vi "GEOM_ReadDetector.vi"(6 "override format":string, 8 "error in (no error)":errorcluster, 9 "detectors path":path=path "/home/ArcVIEW/Modules/Geometry/database", 10 "Detector Name":string, 11 "database path":path=path "/home/ArcVIEW/Modules/Geometry/database") -> (0 "error out":errorcluster, 2 "Detector":T6 {"ReadModes"."amplifiers"."fliped" items=["none", "horizontal", "vertical"]; "ReadModes"."amplifiers"."type" items=["LL", "LR", "UL", "UR"]}, 3 "file path out":path=path "/home/ArcVIEW/Modules/Geometry/database/TYPES/Hawaii-II_4ch.chp", 5 "ydata":i32, 7 "xdata":i32)   [LabVIEW 2016]
uses:
  GEOM_ReadMode.ctl
  GEOM_Amplifier.ctl
  GEOM_AmpType.ctl
  GEOM_ROI.ctl
  GEOM_Coords.ctl
panel:
  in  "ReadMode":T1 {"amplifiers"."fliped" items=["none", "horizontal", "vertical"]; "amplifiers"."type" items=["LL", "LR", "UL", "UR"]}
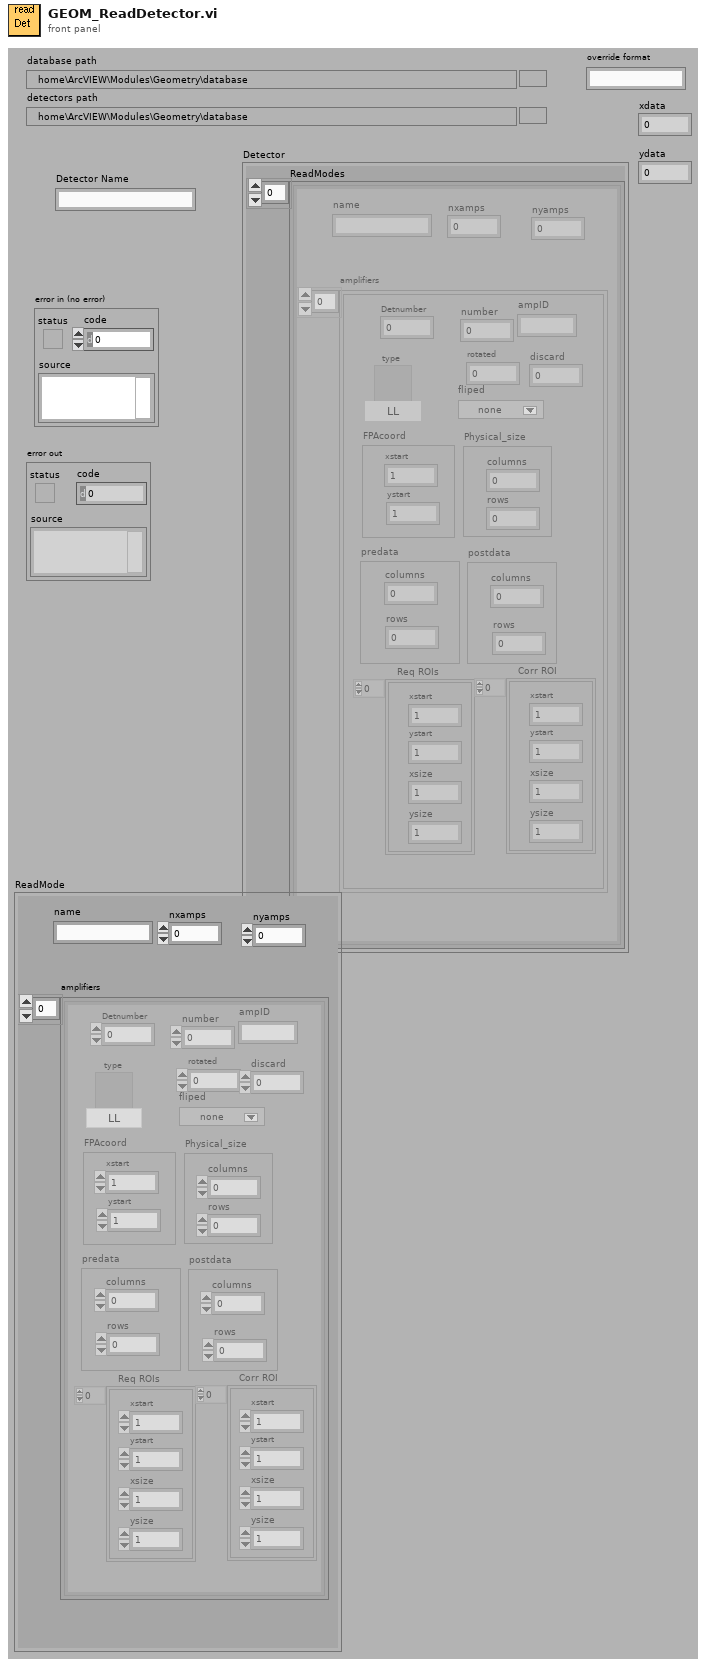
[diagram p1: front panel]
types:
  T1 = typedef "GEOM_ReadMode.ctl" = cluster{"name":string, "amplifiers":T2[], "nxamps":i32, "nyamps":i32}
  T2 = typedef "GEOM_Amplifier.ctl" = cluster{"number":i32, "type":T3, "rotated":i16, "fliped":u16, "FPAcoord":cluster{"xstart":i32, "ystart":i32}, "Physical_size":cluster{"columns":i32, "rows":i32}, "predata":cluster{"columns":i32, "rows":i32}, "postdata":cluster{"columns":i32, "rows":i32}, "Req ROIs":T4, "Corr ROI":T4, "Detnumber":i32, "ampID":string, "discard":i32}
  T3 = typedef "GEOM_AmpType.ctl" = u16
  T4 = typedef "GEOM_ROI.ctl" = T5[]
  T5 = typedef "GEOM_Coords.ctl" = cluster{"xstart":u32, "ystart":u32, "xsize":u32, "ysize":u32}
  T6 = cluster{"name":string, "Info":string[][], "ReadModes":T1[]}
  T7 = cluster{"Detector Name":string, "Info":string[][], "ReadModes":T1[]}
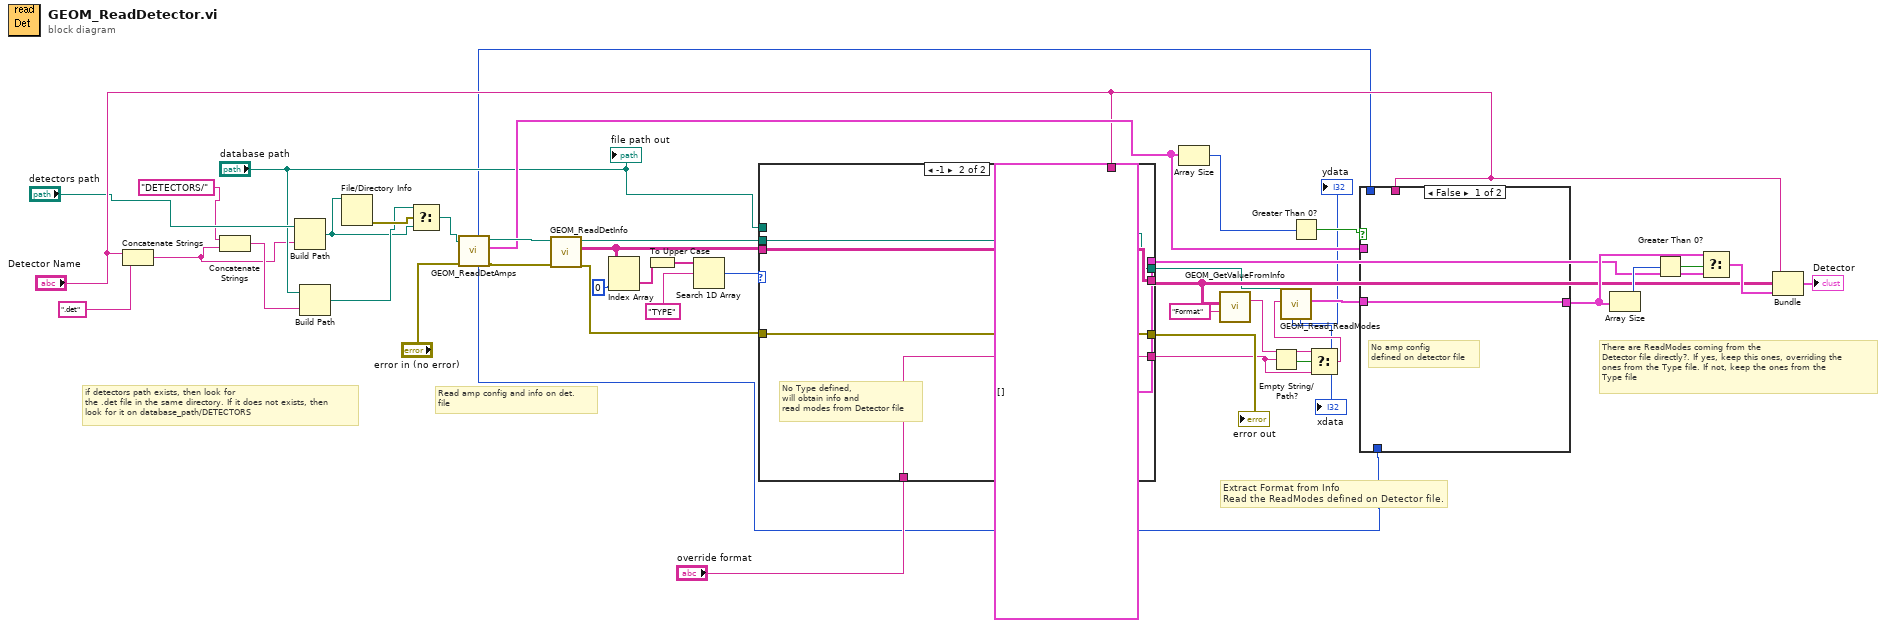
[diagram p0: block diagram]
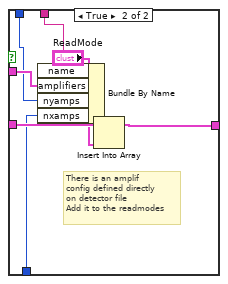
[diagram p2: hidden frame]
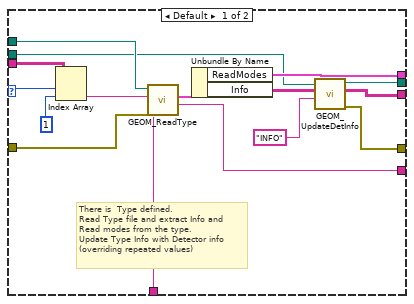
[diagram p3: hidden frame]
diagram:
  # "if detectors path exists, then look for \nthe .det file in the same directory. If it does not exists, then\nlook for it on database_path/DETECTORS"
  # "There are ReadModes coming from the\nDetector file directly?. If yes, keep this ones, overriding the \nones from the Type file. If not, keep the ones from the\nType file"
  # "Extract Format from Info\nRead the ReadModes defined on Detector file."
  # "Read amp config and info on det.\nfile"
  n1 = Concatenate Strings("Detector Name", ".det" ("string")) -> (w4:string)
  n2 = Concatenate Strings("DETECTORS/" ("string"), w4) -> (w5:string)
  n3 = Build Path(base path="detectors path", name or relative path=w4) -> (appended path=w8:path)
  n4 = Build Path(base path="database path", name or relative path=w5) -> (appended path=w9:path)
  n5 = File/Directory Info(path=w8) -> (error out=w12:errorcluster)  [unwired: 1 in, 6 out]
  n6 = Select(t=w9, s=w12, f=w8) -> (s? t:f=w10:path)
  n7 = call "GEOM_ReadDetAmps.vi"("error in (no error)"="error in (no error)", "file path"=w10) -> ("error out"=w36:errorcluster, "amplifiers"=w31:T2[], "cofile path out"=w35:path, "numxamps"=w2:i32, "numyamps"=w3:i32)  [unwired: 2 in, 3 out]
  n8 = call "GEOM_ReadDetInfo.vi"("error in (no error)"=w36, "file path"=w35) -> ("error out"=w41:errorcluster, "Info"=w38:string[][], "file path out"=w7:path)  [unwired: 7 out]
  n9 = Index Array(array=w38, index (col)=0 ("disabled index (col)")) -> (element=w44:string[])  [unwired: 1 in]
  n10 = To Upper Case(1:w44) -> (0:w39:string[])
  n11 = Search 1D Array(1D array=w39, element="TYPE") -> (index of element=w42:i32)  [unwired: 1 out]
  n12 = case shown="-1" w42 {
    selector: w42 -> [w61 _]
    tunnel: w41 -> [w58 w65]
    tunnel: [w55 w65] -> w40
    tunnel: [w54 w66] -> w25
    tunnel: w38 -> [w59 w66]
    tunnel: "database path" -> [w49 _]
    tunnel: [w52 T1[] [] ("ReadModes")] -> w27
    tunnel: [w47 w63] -> w20
    tunnel: "Detector Name" -> [_ _]
    tunnel: "override format" -> [w50 w62]
    tunnel: w7 -> [w48 w63]
    tunnel: [w46 w62] -> w1
    frame Default {
      # "There is  Type defined.\nRead Type file and extract Info and\nRead modes from the type.\nUpdate Type Info with Detector info\n(overriding repeated values)"
      n13 = Index Array(array=w59, index (row)=w61, index (col)=1 ("disabled index (col)")) -> (element=w51:string)
      n14 = call "GEOM_ReadType.vi"("override format"=w50, "error in (no error)"=w58, "TYPE"=w51, "database path"=w49) -> ("format out"=w46:string, "Detector"=w57:cluster{"Info":string[][], "ReadModes":T1[]})  [unwired: 6 out]
      n15 = Unbundle By Name(w57) -> ("ReadModes"=w52:T1[], "Info"=w53:string[][])
      n16 = call "GEOM_UpdateDetInfo.vi"("section"="INFO", "Info In"=w53, "configuration file path"=w48) -> ("error out"=w55:errorcluster, "Info Out"=w54:string[][], "file path out"=w47:path)  [unwired: 1 in, 5 out]
    }
    frame -1 {
      # "No Type defined,\nwill obtain info and\nread modes from Detector file"
    }
  }
  "error out" <- w40
  n17 = Array Size(array=w31) -> (size(s)=w34:i32)
  n18 = call "GEOM_GetValueFromInfo.vi"("Key"="Format", "Info"=w25) -> ("Value"=w18:string)  [unwired: 9 out]
  n19 = Empty String/Path?(string/path=w1) -> (empty?=w19:bool)
  n20 = Greater Than 0?(x=w34) -> (x > 0?=w33:bool)
  n21 = Select(t=w18, s=w19, f=w1) -> (s? t:f=w17:string)
  n22 = call "GEOM_Read_ReadModes.vi"("Detector Format"=w17, "file path"=w20) -> ("ReadModes"=w32:T1[], "ydata"=→"ydata":i32, "xdata"=→"xdata":i32)  [unwired: 1 in, 6 out]
  n23 = case shown="False" w33 {
    tunnel: w32 -> [w67 w75]
    tunnel: w31 -> [_ w71]
    tunnel: "Detector Name" -> [_ w70]
    tunnel: [w67 w73] -> w28
    tunnel: w3 -> [_ w68]
    tunnel: w2 -> [_ w69]
    frame False {
      # "No amp config\ndefined on detector file"
    }
    frame True {
      # "There is an amplif\nconfig defined directly\non detector file\nAdd it to the readmodes"
      n24 = Bundle By Name(cluster="ReadMode", "name"=w70, "amplifiers"=w71, "nyamps"=w68, "nxamps"=w69) -> (w74:T1)
      n25 = Insert Into Array(array=w75, new element=w74) -> (w73:T1[])  [unwired: 1 in]
    }
  }
  n26 = Array Size(array=w28) -> (size(s)=w29:i32)
  n27 = Greater Than 0?(x=w29) -> (x > 0?=w30:bool)
  n28 = Select(t=w28, s=w30, f=w27) -> (s? t:f=w26:T1[])
  n29 = Bundle("Detector Name"="Detector Name", "Info"=w25, "ReadModes"=w26) -> (→"Detector":T7)  [unwired: 1 out]
  "file path out" <- "database path"
